vi "Destroy.vi"(0 "reference in":refnum<class "Customers.lvclass">, 5 "error in (no error)":errorcluster) -> (14 "reference out":refnum<class "Customers.lvclass">, 19 "error out":errorcluster)   [LabVIEW 2020, in "Customers.lvclass"]
uses:
  Customers.lvclass
  CustomersBase_class/CustomersBase.lvclass
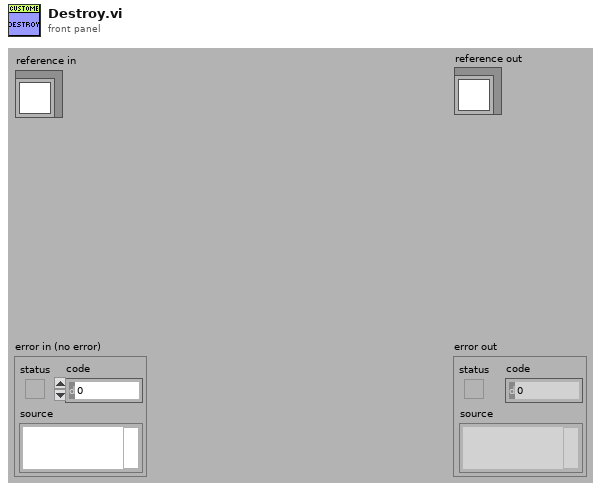
[diagram p1: front panel]
types:
  T1 = typedef "Customers.lvclass/ObjectAttributes.ctl" = cluster{"None":bool}
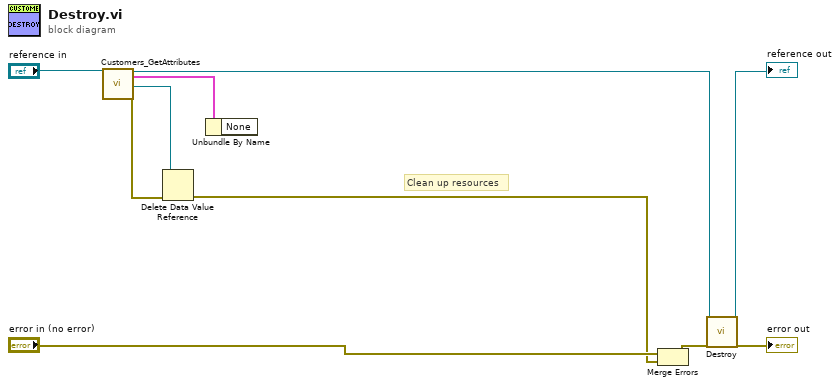
[diagram p0: block diagram]
diagram:
  # "Clean up resources"
  n1 = call "Customers_GetAttributes.vi"("reference in"="reference in") -> ("reference out"=w4:refnum<class "Customers.lvclass">, "Data"=w7:T1, "DataRef"=w8:refnum<data-value>, "error out"=w9:errorcluster)  [unwired: 15 in]
  n2 = Delete Data Value Reference(data value reference=w8, error in=w9) -> (error out=w1:errorcluster)  [unwired: 1 out]
  n3 = Unbundle By Name(w7) -> ()  [unwired: 1 out]
  n4 = Merge Errors("error in (no error)", w1) -> (w6:errorcluster)
  n5 = call-parent "Destroy.vi"("reference in"=w4, "error in (no error)"=w6) -> ("reference out"=→"reference out":refnum<class "Customers.lvclass">, "error out"=→"error out":errorcluster)  [unwired: 16 in]
